vi "RD Digital SPI Tx Rx IO Set.vi"(6 "DQ1":i32, 7 "DQ0":i32, 8 "error in (no error)":errorcluster caption="错误输入（无错误）", 9 "ClockDIO":i32, 10 "CSDIO":i32, 11 "handle":u64) -> (0 "error out":errorcluster caption="错误输出", 2 "function return":i32, 3 "handle out":u64)   [LabVIEW 2018, in "InstrumentsPlayground.lvlib"]
doc: "CLIFFAPI int CliffDigitalSPIRateSet(FT_HANDLE handle, double rate); CLIFFAPI int CliffDigitalSPITxRxIOSet(FT_HANDLE handle, int TxDIO,int RxDIO,int DQ0, int DQ1);"
uses:
  InstrumentsPlayground.lvlib
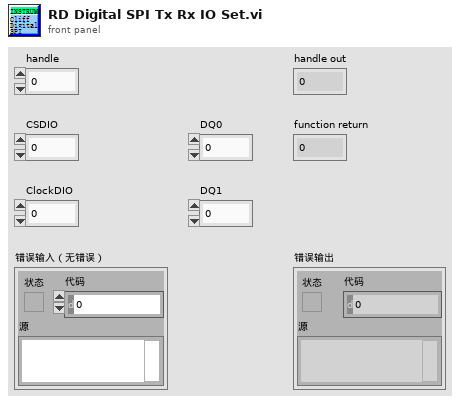
[diagram p1: front panel]
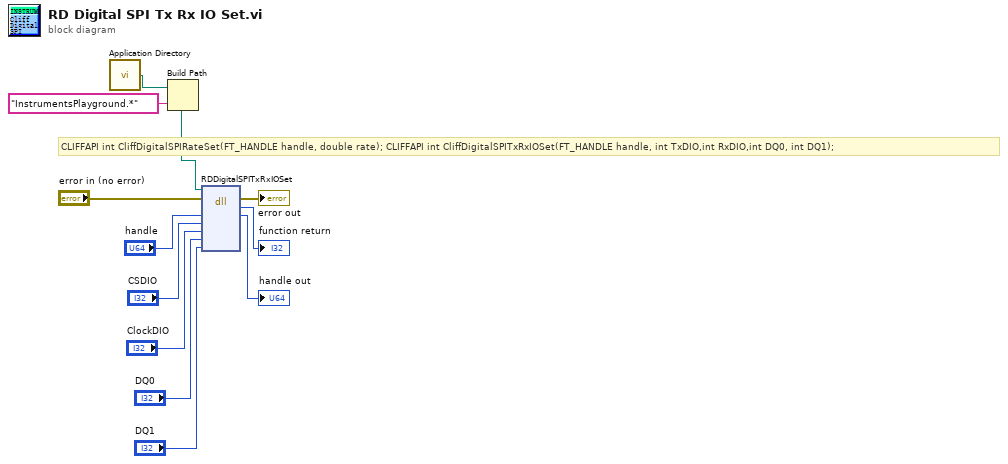
[diagram p0: block diagram]
diagram:
  # "CLIFFAPI int CliffDigitalSPIRateSet(FT_HANDLE handle, double rate); CLIFFAPI int CliffDigitalSPITxRxIOSet(FT_HANDLE handle, int TxDIO,int RxDIO,int DQ0, int DQ1);"
  n1 = call <vilib>:"Application Directory.vi"() -> ("Application Directory"=w2:path)
  n2 = Build Path(base path=w2, name or relative path="InstrumentsPlayground.*" ("名称或相对路径")) -> (appended path=w1:path)
  n3 = dll-call lib="E:/Work/YZCourse_Xtext/Cliff/API/IPLabView lib/InstrumentsPlayground.*" fn="RDDigitalSPITxRxIOSet"(path in=w1, error in="error in (no error)", "handle"="handle", "CSDIO"="CSDIO", "ClockDIO"="ClockDIO", "DQ0"="DQ0", "DQ1"="DQ1") -> (error out=→"error out":errorcluster, "返回类型"=→"function return":i32, "handle"=→"handle out":u64)  [unwired: 5 in, 1 out]
